vi "Memory.Pointer.Error Handler.Out of Bounds.vi"(8 "error in (no error)":errorcluster, 10 "length (0)":i64 format="%d bytes", 11 "offset (0)":i64 format="%d bytes") -> (0 "error out":errorcluster)   [LabVIEW 2016, in "LabVIEW Memory Manager.lvlib" / "Memory.Pointer.lvclass"]
uses:
  Memory.Pointer.lvclass
  Typedefs/Memory.Pointer.Error Codes.ctl
  LabVIEW Memory Manager.lvlib
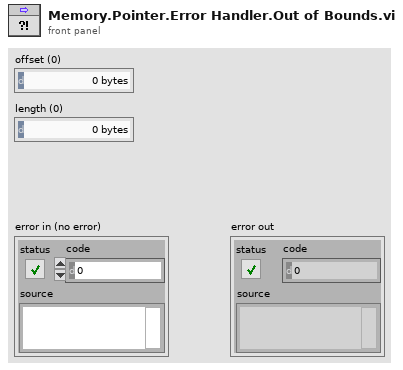
[diagram p1: front panel]
types:
  T1 = typedef "LabVIEW Memory Manager.lvlib/Memory.Pointer.lvclass/Memory.Pointer.Error Codes.ctl" = i32
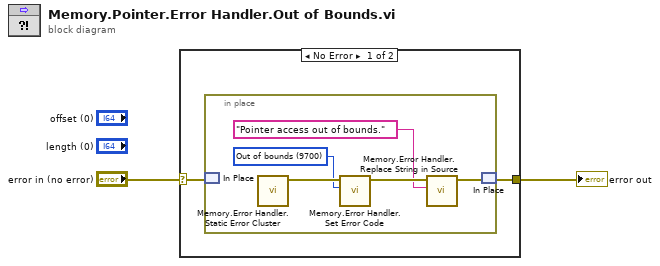
[diagram p0: block diagram]
diagram:
  n1 = case shown="No Error" "error in (no error)" {
    selector: "error in (no error)" -> [w4 w10]
    tunnel: [w3 w10] -> w1
    frame No Error {
      n2 = in-place {
        w7 = T1 9700 items=["Out of bounds"=9700] ("Pointer error code")
        n3 = in-place-match #1(w4) -> ()  [unwired: 1 out]
        n4 = call "Memory.Error Handler.Static Error Cluster.vi"() -> ("error out"=w9:errorcluster)  [unwired: 11 in]
        n5 = call "Memory.Error Handler.Set Error Code.vi"("code"=w7, "error in"=w9) -> ("error out"=w8:errorcluster)  [unwired: 9 in]
        n6 = call "Memory.Error Handler.Replace String in Source.vi"("string"="Pointer access out of bounds." ("substring (\"\")"), "error in"=w8) -> ("error out"=w5:errorcluster)  [unwired: 8 in, 1 out]
        n7 = in-place-match #1(w5) -> (w3:errorcluster)
      }
    }
    frame Error {
      # "Error already on wire. Pass through."
    }
  }
  "error out" <- w1
